vi "duplicate.vi"(8 "error in":errorcluster, 11 "configuration in":refnum<class "NISE_CEF_serializable configuration.lvclass">) -> (0 "error out":errorcluster, 2 "duplicate configuration out":refnum<class "NISE_CEF_serializable configuration.lvclass">, 3 "original configuration out":refnum<class "NISE_CEF_serializable configuration.lvclass">)   [LabVIEW 2013, in "NISE_CEF_serializable configuration.lvclass"]
uses:
  NISE_CEF_serializable configuration.lvclass
  NISE_CEF_serializable configuration.lvclass/NISE_CEF_serializable configuration.ctl
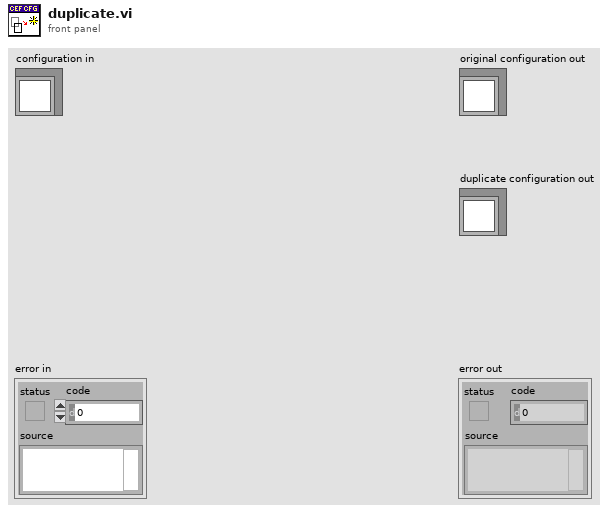
[diagram p1: front panel]
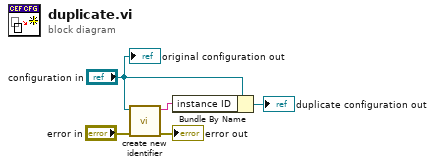
[diagram p0: block diagram]
diagram:
  n1 = call-dynamic "create new identifier.vi"("error in"="error in", "configuration in"="configuration in") -> ("error out"=→"error out":errorcluster, "id"=w3:string)  [unwired: 8 in]
  n2 = Bundle By Name(cluster="configuration in", "instance ID"=w3) -> (→"duplicate configuration out":refnum<class "NISE_CEF_serializable configuration.lvclass">)
  "original configuration out" <- "configuration in"
